vi "Wavelet Transform and Reconstruction with Image.vi"() -> ()   [LabVIEW 2023]
doc: "This example shows how to perform image decomposition and reconstruction with the WA Discrete Wavelet Transform VI and the WA Inverse Discrete Wavelet Transform VI, respectively.\n\n<b>Instructions:</b>\n1) Run this VI.\n2) Browse the Block Diagram of this example to learn how to perform image decomposition and reconstruction by using the 2D discrete wavelet decomposition and reconstruction."
uses:
  <vilib>/addons/Wavelet Analysis/discrete wavelet transform.llb/WA 2D Discrete Wavelet Transform.vi
  <vilib>/addons/Wavelet Analysis/discrete wavelet transform.llb/WA Inverse 2D Discrete Wavelet Transform.vi
  <vilib>/addons/_Advanced Signal Processing/NI_AdvSigProcWA.lvlib
panel:
  in  "Image to show":u16(ring)=122 items=["1D Example Data"=100, "-"=101, "Doppler"=102, "HOP"=103, "TF Sine"=104, "Noisy Doppler"=105, "Sea Temperature"=106, "Sp500"=107, "Power Line"=108, "Engine Knocking"=109, "HeaviSine"=110, "Bumps"=111, "Blocks"=112, "Piece Regular"=113, "HypChirps"=114, "LinChirps"=115, "Chirps"=116, "Piece Polynomial"=117, "ECG"=131, "-"=118, "2D Example Data"=119, "-"=120, "Finger Print (Image)"=121, "Iris Flower (Image)"=122, "Mammogram (Image)"=123, "Lake (Image)"=127, "Two Can 1 (Image)"=132, "Two Can 2 (Image)"=133, "Camera Man (Image)"=134]
  in  "Levels":i32=8
  in  "Wavelet":u16(ring) items=["db02"=0, "db03"=1, "db04"=2, "db05"=3, "db06"=4, "db07"=5, "db08"=6, "db09"=7, "db10"=8, "db11"=9, "db12"=10, "db13"=11, "db14"=12, "Haar"=13, "bior1_3"=14, "bior1_5"=15, "bior2_2"=16, "bior2_4"=17, "bior2_6"=18, "bior2_8"=19, "bior3_1"=20, "bior3_3"=21, "bior3_5"=22, "bior3_7"=23, "bior3_9"=24, "bior4_4 (FBI)"=25, "bior5_5"=38, "bior6_8"=39, "coif1"=26, "coif2"=27, "coif3"=28, "coif4"=29, "coif5"=30, "sym2"=31, "sym3"=32, "sym4"=33, "sym5"=34, "sym6"=35, "sym7"=36, "sym8"=37]
  out "Reconstructed Image":dbl[][](graph)
  out "Image":u8[][](graph)
  # "Overview: Shows how to perform image decomposition and reconstruction with the WA Discrete Wavelet Transform VI and the WA Inverse Discrete Wavelet Transform VI, respectively.\nRequirements: LabVIEW Full Development System, Advanced Signal Processing Toolkit\nInstructions: \n1. Run this VI.\n2. Browse the block diagram of this example to learn how to perform image decomposition and reconstruction by using the 2D discrete wavelet decomposition and reconstruction."
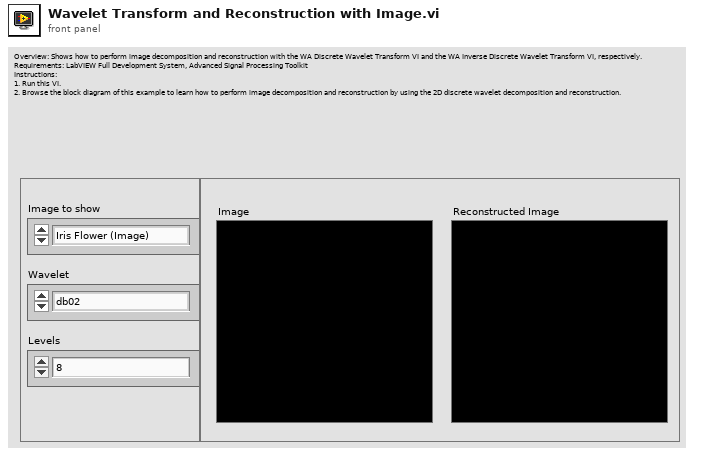
[diagram p1: front panel]
types:
  T1 = cluster{"low_low":dbl[][], "low_high":dbl[][], "high_low":dbl[][], "high_high":dbl[][]}[]
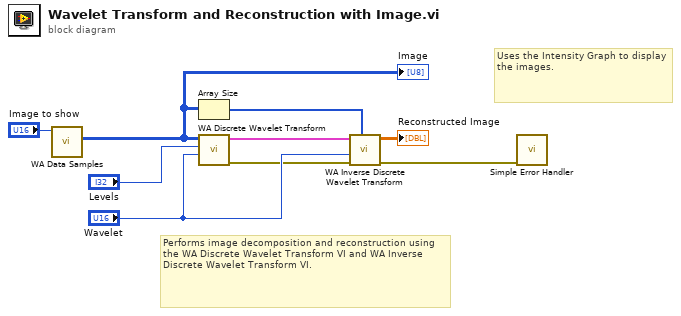
[diagram p0: block diagram]
diagram:
  # "Uses the Intensity Graph to display the images."
  # "Performs image decomposition and reconstruction using the WA Discrete Wavelet Transform VI and WA Inverse Discrete Wavelet Transform VI."
  n1 = call <vilib>:"WA Data Samples.vi"("data"="Image to show") -> ("image"=w4:u8[][])  [unwired: 10 out]
  "Image" <- w4
  n2 = Array Size(array=w4) -> (size(s)=w8:i32[])
  n3 = call-poly <vilib>:"WA Discrete Wavelet Transform.vi"("wavelet"="Wavelet", "levels"="Levels", "signal"=w4) -> ("error out"=w2:errorcluster, "DWT coef"=w5:T1)  [unwired: 1 in, 6 out]
  n4 = call-poly <vilib>:"WA Inverse Discrete Wavelet Transform.vi"("size"=w8, "error in (no error)"=w2, "wavelet"="Wavelet", "DWT coef"=w5) -> ("error out"=w1:errorcluster, "signal"=→"Reconstructed Image":dbl[][])  [unwired: 6 out]
  n5 = call <vilib>:"Simple Error Handler.vi"("error in (no error)"=w1) -> ()  [unwired: 4 in, 5 out]
